vi "live_edited3.vi"() -> ()   [LabVIEW 2020]
uses:
  C:/Users/Public/Documents/Photometrics/PMQI-LabViewSamples/Examples/2018/Dependencies/PVCamNET.dll
  Dependencies/PVCamNET.dll
panel:
  in  "Full CCD Height":u16
  in  "Full CCD Width":u16
  in  "Full CCD":bool
  in  "Get ROI":bool
  in  "Height":u16
  in  "Y":u16
  in  "Width":u16
  in  "X":u16
  out "Trigger Mode":i32
  in  "Trigger In Behaviour":string(combo)
  out "Exp. out":i32
  in  "Trigger Out Behaviour":string(combo)
  out "Boolean":bool
  in  "Scan Direction Reset":bool
  out "Scan Line Time":dbl format="%#_14g"
  in  "Scan Width":dbl
  in  "Scan Line Delay":dbl
  in  "Scan Direction":string(combo)
  in  "Scan Mode":string(combo)
  in  "Exposure Time":dbl
  in  "Live":bool
  in  "Camera Status":bool
  in  "Uninit":bool
  in  "Live stop":bool
  in  "Live start":bool
  in  "Open":bool
  # "Description:\nThis code lets the user use programmable scan\n mode for live imaging.\n\nSteps to run:\n1. Click \"Run\"\n2. Click \"Open\"\n3. Enter Exposure Time\n4. Select Scan Mode. \n5. Set Scan Line Delay or Scan Width\n6. Select Scan Direction\n7. Click \"Live start\"\n8. Click \"Live stop\"\n9. Right click on CamWindow and add a ROI.\n10. Click \"Get ROI\"\n11. Click \"Live start\"\n12. Click \"Live stop\"\n13. Right click on CamWindow and delete a ROI.\n14. Click \"Close\""
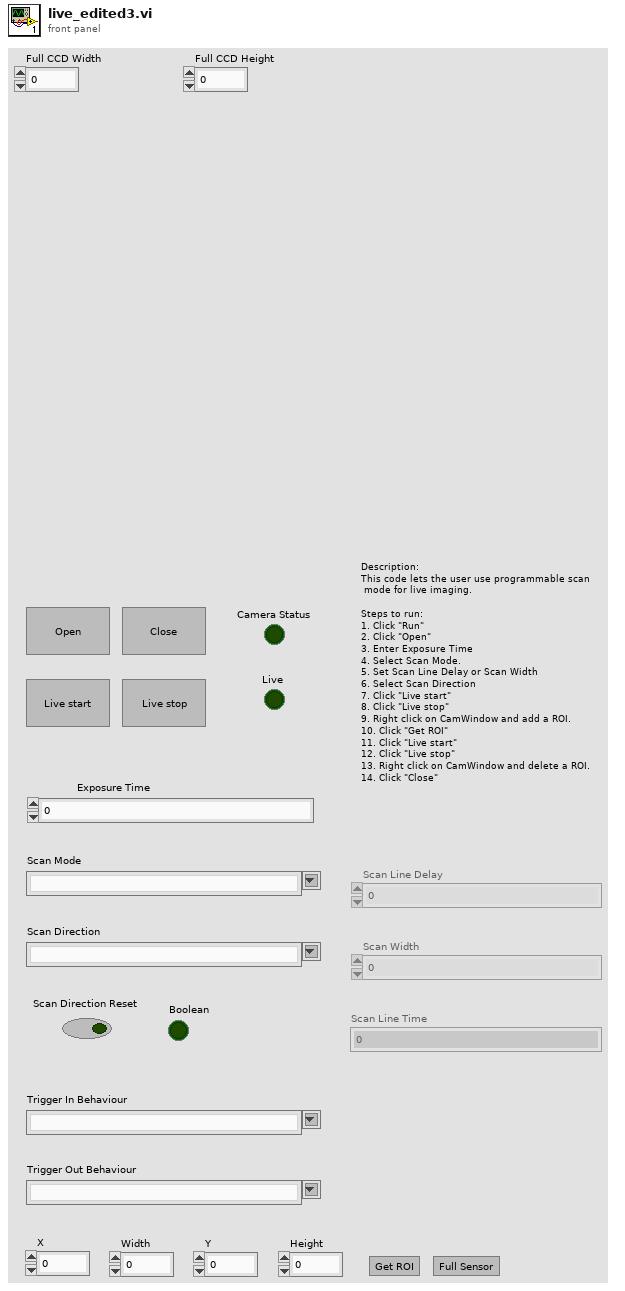
[diagram p1: front panel]
types:
  T1 = enum8{"Enabled", "Disabled", "Disabled and Grayed Out"}
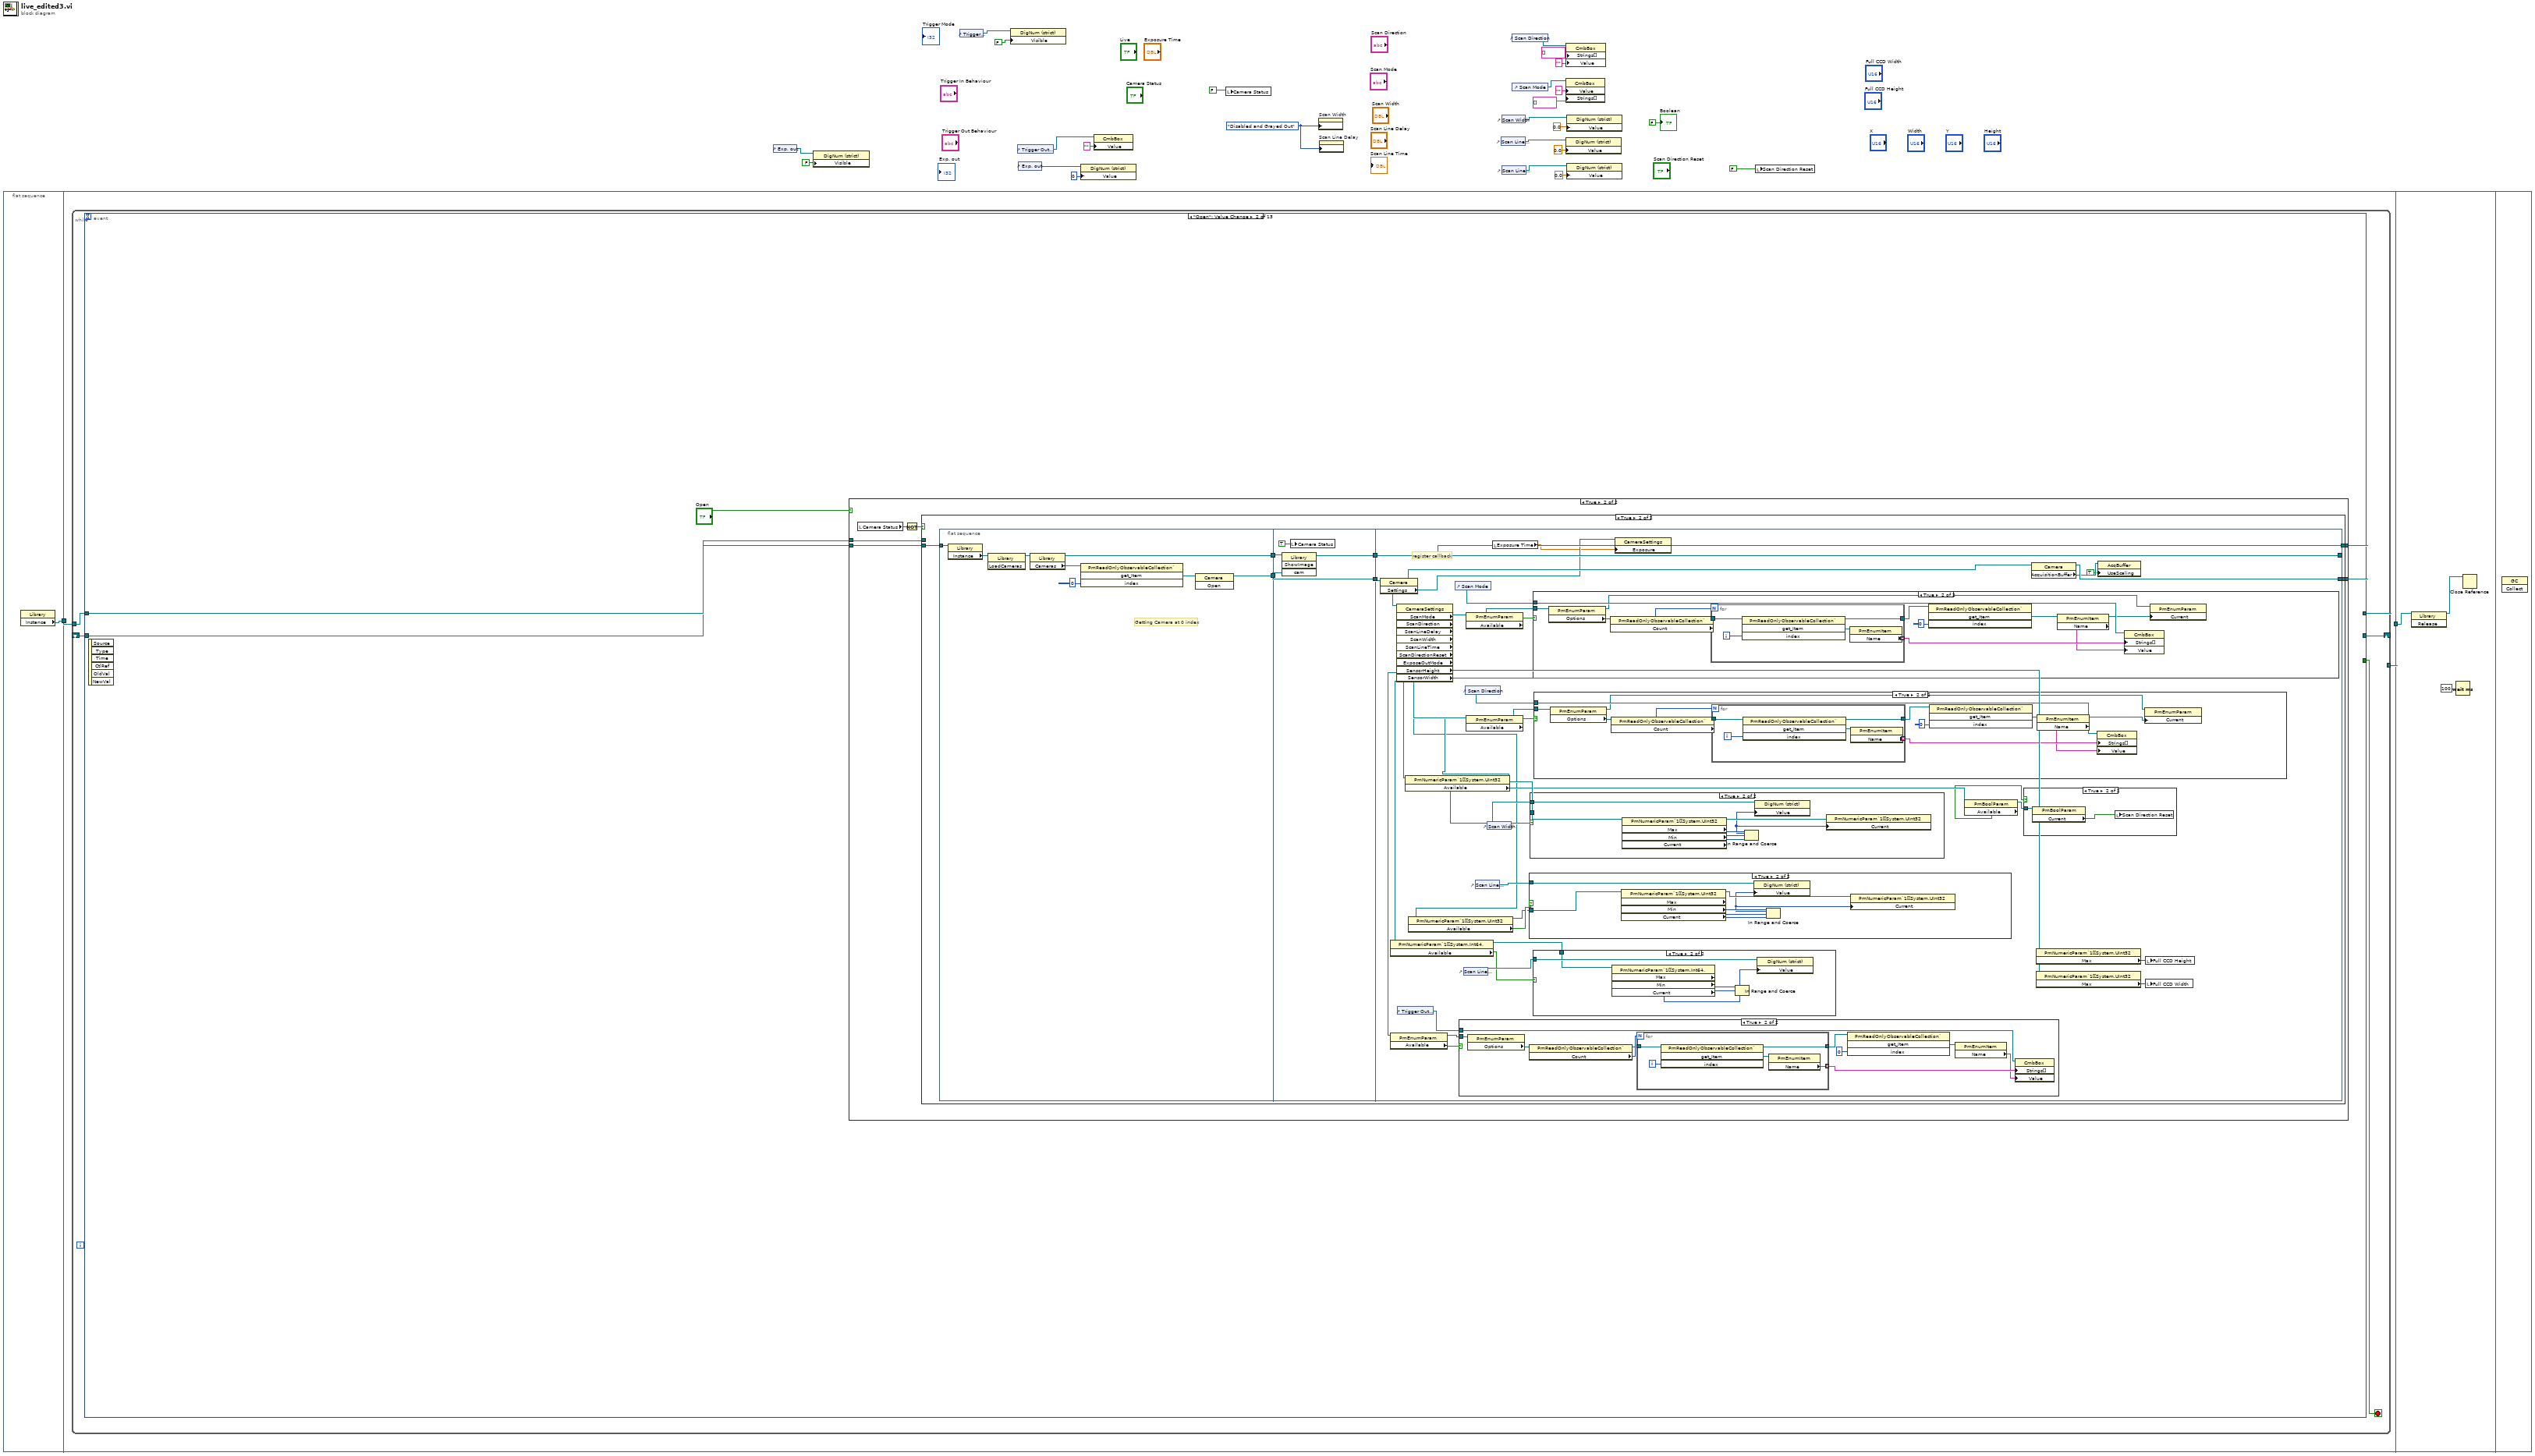
[diagram p0: block diagram]
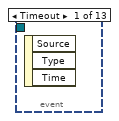
[diagram p2: hidden frame]
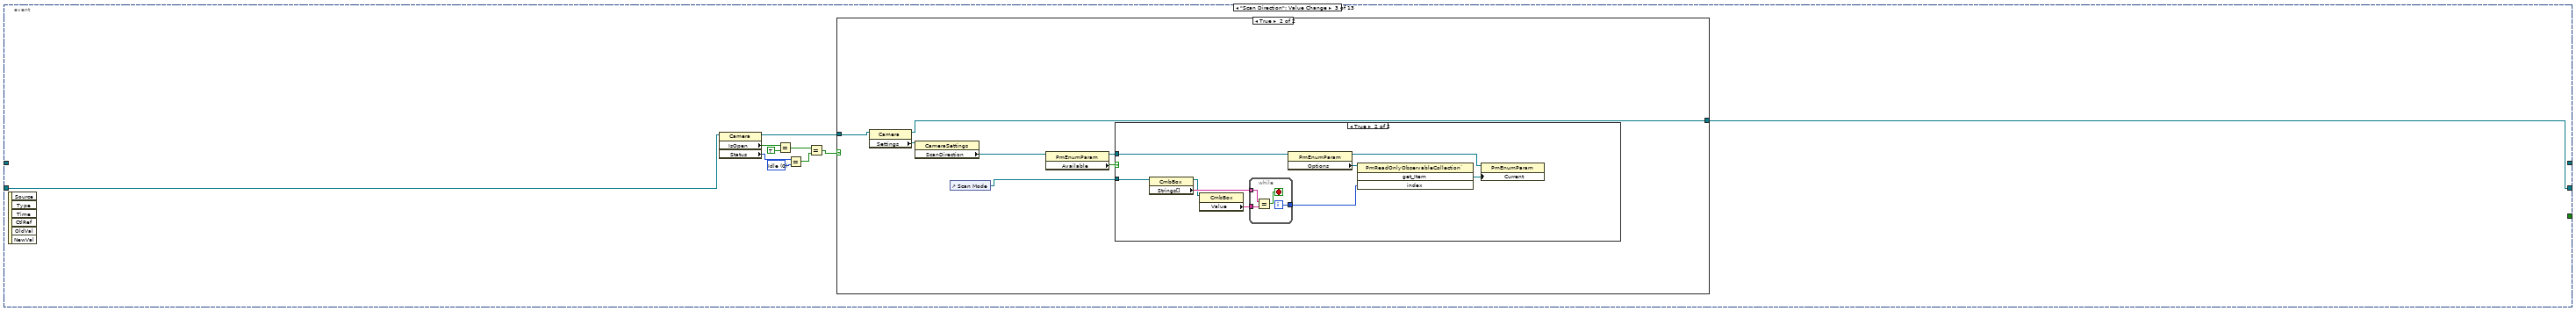
[diagram p12: hidden frame]
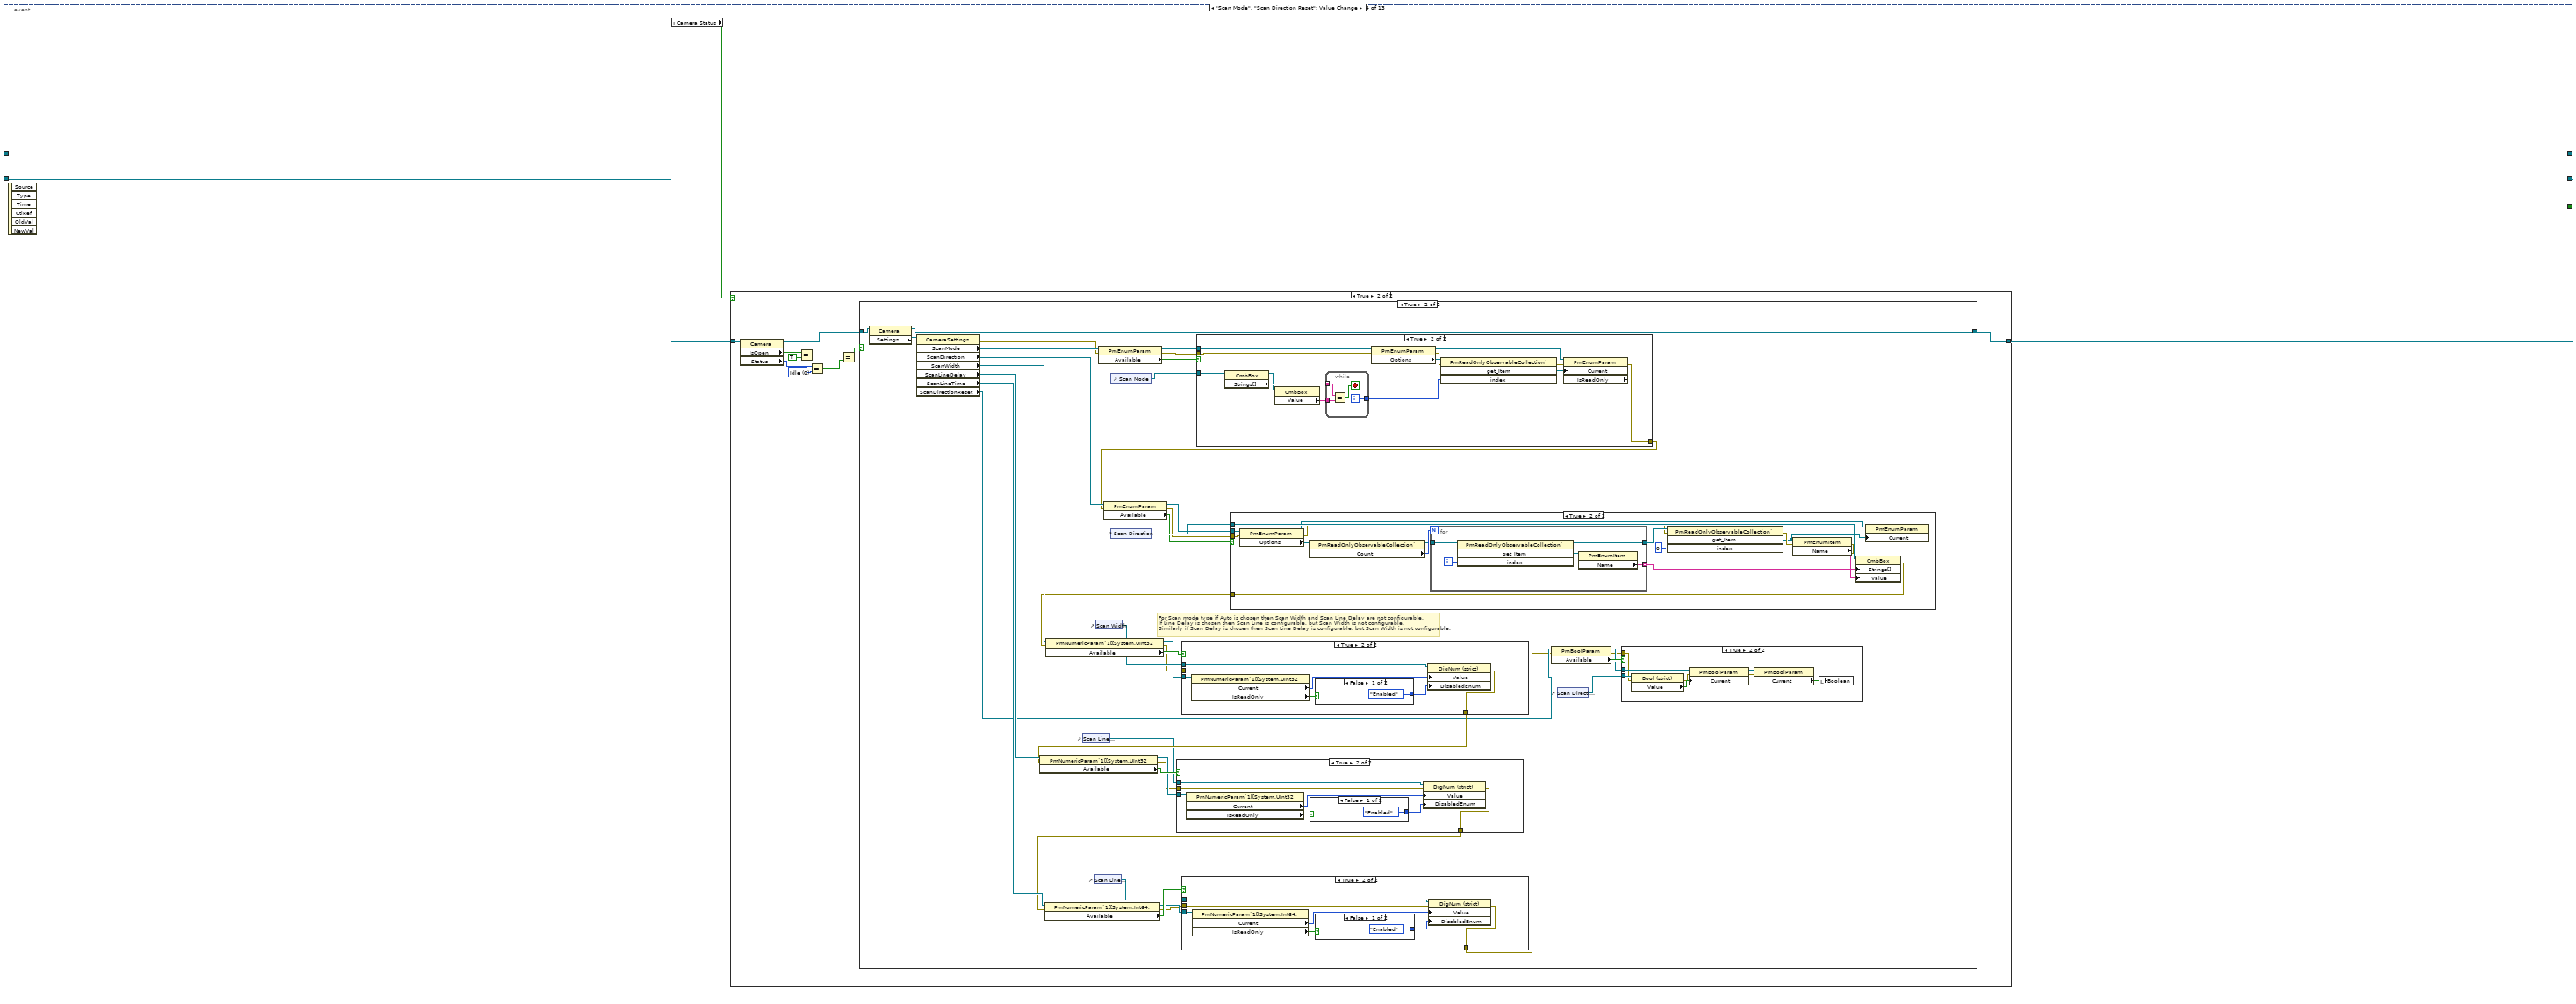
[diagram p15: hidden frame]
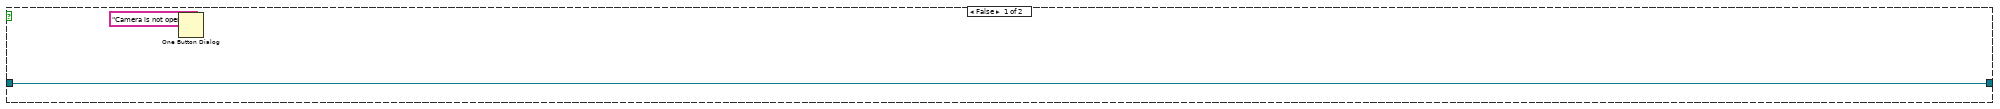
[diagram p16: hidden frame]
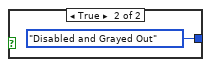
[diagram p20: hidden frame]
diagram:
  w11 = T1."Disabled and Grayed Out" ("Disabled")
  n1 = flat-sequence {
    tunnel: [w27] -> w26
    tunnel: w26 -> [w29]
    tunnel: [w28] -> w25
    tunnel: w25 -> [w765]
    frame #0 {
      n2 = property class="Library"() -> ("Instance"=w27:refnum<k24>)  [unwired: 2 in, 2 out]
    }
    frame #1 {
      n3 = while {
        tunnel: w29 -> [w34]
        shift-right: [w33] -> _
        shift-left: _ -> [w31]
        tunnel: [w32] -> w28
        stop <- w30 stop-if-true
        n4 = event shown="[1] \"Open\": Value Change" {
          selector: _ -> [_ _ _ _ _ _ _ _ _ _ _ _ _]
          dyn-events: _ -> [_ _ _ _ _ _ _ _ _ _ _ _ _]
          timeout: _ -> [_ _ _ _ _ _ _ _ _ _ _ _ _]
          tunnel: w34 -> [_ w39 _ _ _ _ w466 _ _ _ w682 _ w737]
          tunnel: [_ w38 w179 w211 w343 w407 w467 w534 w571 w644 w683 w712 w738] -> w33
          tunnel: [_ w37 _ _ _ _ w466 _ _ _ w682 _ w737] -> w32
          tunnel: w31 -> [_ w36 w183 w212 w349 w409 w468 w535 w572 w645 w684 w713 w739]
          tunnel: [_ _ _ _ _ _ _ _ _ _ _ _ w736] -> w30
          event Timeout {
            n5 = event-data() -> ()  [unwired: 1 in, 3 out]
          }
          event "Open": Value Change {
            n6 = event-data() -> ()  [unwired: 1 in, 6 out]
            n7 = case shown="True" "Open" {
              tunnel: w39 -> [w41 w47]
              tunnel: [w40 w46] -> w38
              tunnel: [w41 w45] -> w37
              tunnel: w36 -> [w40 w42]
              frame False {
              }
              frame True {
                n8 = local read "Camera Status"() -> (w44:bool)
                n9 = Not(x=w44) -> (.not. x?=w43:bool)
                n10 = case shown="True" w43 {
                  tunnel: w47 -> [w48 w54]
                  tunnel: [w49 w53] -> w46
                  tunnel: [w48 w52] -> w45
                  tunnel: w42 -> [w49 _]
                  frame False {
                  }
                  frame True {
                    n11 = flat-sequence {
                      tunnel: w54 -> [w59]
                      tunnel: [w61] -> w56
                      tunnel: [w60] -> w55
                      tunnel: w56 -> [w67]
                      tunnel: w55 -> [w68]
                      tunnel: [w68] -> w51
                      tunnel: [w66] -> w50
                      tunnel: [w107] -> w52
                      tunnel: [w87] -> w53
                      tunnel: w51 -> [w106]
                      tunnel: w50 -> [w107]
                      frame #0 {
                        # "Getting Camera at 0 index"
                        n12 = property class="Library"(reference=w59) -> ("Instance"=w58:refnum<k24>)  [unwired: 1 in, 2 out]
                        n13 = invoke class="Library" method="LoadCameras"(reference=w58) -> (reference out=w57:refnum<k24>)  [unwired: 2 in, 2 out]
                        n14 = property class="Library"(reference=w57) -> (reference out=w61:refnum<k24>, "Cameras"=w64:refnum<k24>)  [unwired: 1 in, 1 out]
                        n15 = invoke class="PmReadOnlyObservableCollection`" method="get_Item"(reference=w64, "index"=0) -> ("get_Item"=w62:refnum<k24>)  [unwired: 2 in, 3 out]
                        n16 = invoke class="Camera" method="Open"(reference=w62) -> (reference out=w60:refnum<k24>)  [unwired: 2 in, 2 out]
                      }
                      frame #1 {
                        n17 = invoke class="Library" method="ShowImage"(reference=w67, "cam"=w68) -> (reference out=w66:refnum<k24>)  [unwired: 2 in, 3 out]
                        n18 = local write "Camera Status"(TRUE ("Camera Status")) -> ()
                      }
                      frame #2 {
                        # "register callback"
                        n19 = property class="Camera"(reference=w106) -> (reference out=w88:refnum<k24>, "Settings"=w77:refnum<k24>)  [unwired: 1 in, 1 out]
                        n20 = property class="CameraSettings"(reference=w77) -> ("ScanMode"=w105:refnum<k24>, "ScanDirection"=w101:refnum<k24>, "ScanLineDelay"=w96:refnum<k24>, "ScanWidth"=w83:refnum<k24>, "ScanLineTime"=w75:refnum<k24>, "ScanDirectionReset"=w91:refnum<k24>, "ExposeOutMode"=w79:refnum<k24>, "SensorHeight"=w70:refnum<k24>, "SensorWidth"=w69:refnum<k24>)  [unwired: 1 in, 2 out]
                        n21 = property class="PmNumericParam`1[[System.Int64,"(reference=w75) -> (reference out=w73:refnum<k24>, "Available"=w74:bool)  [unwired: 1 in, 1 out]
                        n22 = property class="PmEnumParam"(reference=w79) -> (reference out=w80:refnum<k24>, "Available"=w81:bool)  [unwired: 1 in, 1 out]
                        n23 = control-ref of="Trigger Out Behaviour"() -> (w78:refnum<vi>)
                        n24 = property class="PmNumericParam`1[[System.UInt32"(reference=w96) -> (reference out=w94:refnum<k24>, "Available"=w95:bool)  [unwired: 1 in, 1 out]
                        n25 = property class="PmNumericParam`1[[System.UInt32"(reference=w83) -> (reference out=w82:refnum<k24>, "Available"=w84:bool)  [unwired: 1 in, 1 out]
                        n26 = control-ref of="Scan Mode"() -> (w102:refnum<vi>)
                        n27 = case shown="True" w81 {
                          tunnel: w80 -> [_ w117]
                          tunnel: w78 -> [_ w108]
                          frame False {
                          }
                          frame True {
                            n28 = property class="PmEnumParam"(reference=w117) -> ("Options"=w116:refnum<k24>)  [unwired: 1 in, 2 out]
                            n29 = property class="PmReadOnlyObservableCollection`"(reference=w116) -> (reference out=w114:refnum<k24>, "Count"=w115:i32)  [unwired: 1 in, 1 out]
                            n30 = for {
                              N: w115 -> [_]
                              tunnel: w114 -> [w122]
                              tunnel: [w119] -> w111
                              tunnel: [w118] -> w110 mode=indexing
                              i -> [w121]
                              n31 = invoke class="PmReadOnlyObservableCollection`" method="get_Item"(reference=w122, "index"=w121) -> (reference out=w119:refnum<k24>, "get_Item"=w120:refnum<k24>)  [unwired: 2 in, 2 out]
                              n32 = property class="PmEnumItem"(reference=w120) -> ("Name"=w118:string)  [unwired: 1 in, 2 out]
                            }
                            n33 = invoke class="PmReadOnlyObservableCollection`" method="get_Item"(reference=w111, "index"=0) -> ("get_Item"=w112:refnum<k24>)  [unwired: 2 in, 3 out]
                            n34 = property class="PmEnumItem"(reference=w112) -> ("Name"=w109:string)  [unwired: 1 in, 2 out]
                            n35 = property class="CmbBox"(reference=w108, "Strings[]"=w110, "Value"=w109) -> ()  [unwired: 1 in, 2 out]
                          }
                        }
                        n36 = control-ref of="Scan Line Time"() -> (w92:refnum<vi>)
                        n37 = control-ref of="Scan Direction"() -> (w98:refnum<vi>)
                        n38 = property class="PmEnumParam"(reference=w105) -> (reference out=w103:refnum<k24>, "Available"=w104:bool)  [unwired: 1 in, 1 out]
                        n39 = property class="PmEnumParam"(reference=w101) -> (reference out=w99:refnum<k24>, "Available"=w100:bool)  [unwired: 1 in, 1 out]
                        n40 = control-ref of="Scan Line Delay"() -> (w93:refnum<vi>)
                        n41 = control-ref of="Scan Width"() -> (w97:refnum<vi>)
                        n42 = local read "Exposure Time"() -> (w76:dbl)
                        n43 = case shown="True" w84 {
                          tunnel: w93 -> [_ w134]
                          tunnel: w82 -> [_ w133]
                          frame False {
                          }
                          frame True {
                            n44 = property class="PmNumericParam`1[[System.UInt32"(reference=w133) -> (reference out=w132:refnum<k24>, "Max"=w135:u32, "Min"=w136:u32, "Current"=w137:u32)  [unwired: 1 in, 1 out]
                            n45 = In Range and Coerce(upper limit=w135, x=w137, lower limit=w136) -> (coerced(x)=w131:u32)  [unwired: 1 out]
                            n46 = property class="DigNum (strict)"(reference=w134, "Value"=w131) -> ()  [unwired: 1 in, 2 out]
                            n47 = property class="PmNumericParam`1[[System.UInt32"(reference=w132, "Current"=w131) -> ()  [unwired: 1 in, 2 out]
                          }
                        }
                        n48 = case shown="True" w95 {
                          tunnel: w97 -> [_ w141]
                          tunnel: w94 -> [_ w140]
                          frame False {
                          }
                          frame True {
                            n49 = property class="PmNumericParam`1[[System.UInt32"(reference=w140) -> (reference out=w139:refnum<k24>, "Max"=w142:u32, "Min"=w143:u32, "Current"=w144:u32)  [unwired: 1 in, 1 out]
                            n50 = In Range and Coerce(upper limit=w142, x=w144, lower limit=w143) -> (coerced(x)=w138:u32)  [unwired: 1 out]
                            n51 = property class="DigNum (strict)"(reference=w141, "Value"=w138) -> ()  [unwired: 1 in, 2 out]
                            n52 = property class="PmNumericParam`1[[System.UInt32"(reference=w139, "Current"=w138) -> ()  [unwired: 1 in, 2 out]
                          }
                        }
                        n53 = case shown="True" w74 {
                          tunnel: w92 -> [_ w126]
                          tunnel: w73 -> [_ w125]
                          frame False {
                          }
                          frame True {
                            n54 = property class="PmNumericParam`1[[System.Int64,"(reference=w125) -> ("Max"=w127:i64, "Min"=w128:i64, "Current"=w129:i64)  [unwired: 1 in, 2 out]
                            n55 = In Range and Coerce(upper limit=w127, x=w129, lower limit=w128) -> (coerced(x)=w130:i64)  [unwired: 1 out]
                            n56 = property class="DigNum (strict)"(reference=w126, "Value"=w130) -> ()  [unwired: 1 in, 2 out]
                          }
                        }
                        n57 = case shown="True" w104 {
                          tunnel: w103 -> [_ w173]
                          tunnel: w102 -> [_ w165]
                          frame False {
                          }
                          frame True {
                            n58 = property class="PmEnumParam"(reference=w173) -> (reference out=w164:refnum<k24>, "Options"=w172:refnum<k24>)  [unwired: 1 in, 1 out]
                            n59 = property class="PmReadOnlyObservableCollection`"(reference=w172) -> (reference out=w170:refnum<k24>, "Count"=w171:i32)  [unwired: 1 in, 1 out]
                            n60 = for {
                              N: w171 -> [_]
                              tunnel: w170 -> [w178]
                              tunnel: [w175] -> w168
                              tunnel: [w174] -> w167 mode=indexing
                              i -> [w177]
                              n61 = invoke class="PmReadOnlyObservableCollection`" method="get_Item"(reference=w178, "index"=w177) -> (reference out=w175:refnum<k24>, "get_Item"=w176:refnum<k24>)  [unwired: 2 in, 2 out]
                              n62 = property class="PmEnumItem"(reference=w176) -> ("Name"=w174:string)  [unwired: 1 in, 2 out]
                            }
                            n63 = invoke class="PmReadOnlyObservableCollection`" method="get_Item"(reference=w168, "index"=0) -> ("get_Item"=w163:refnum<k24>)  [unwired: 2 in, 3 out]
                            n64 = property class="PmEnumItem"(reference=w163) -> (reference out=w162:refnum<k24>, "Name"=w166:string)  [unwired: 1 in, 1 out]
                            n65 = property class="CmbBox"(reference=w165, "Strings[]"=w167, "Value"=w166) -> ()  [unwired: 1 in, 2 out]
                            n66 = property class="PmEnumParam"(reference=w164, "Current"=w162) -> ()  [unwired: 1 in, 2 out]
                          }
                        }
                        n67 = case shown="True" w100 {
                          tunnel: w99 -> [_ w156]
                          tunnel: w98 -> [_ w147]
                          frame False {
                          }
                          frame True {
                            n68 = property class="PmEnumParam"(reference=w156) -> (reference out=w146:refnum<k24>, "Options"=w155:refnum<k24>)  [unwired: 1 in, 1 out]
                            n69 = property class="PmReadOnlyObservableCollection`"(reference=w155) -> (reference out=w153:refnum<k24>, "Count"=w154:i32)  [unwired: 1 in, 1 out]
                            n70 = for {
                              N: w154 -> [_]
                              tunnel: w153 -> [w161]
                              tunnel: [w158] -> w150
                              tunnel: [w157] -> w149 mode=indexing
                              i -> [w160]
                              n71 = invoke class="PmReadOnlyObservableCollection`" method="get_Item"(reference=w161, "index"=w160) -> (reference out=w158:refnum<k24>, "get_Item"=w159:refnum<k24>)  [unwired: 2 in, 2 out]
                              n72 = property class="PmEnumItem"(reference=w159) -> ("Name"=w157:string)  [unwired: 1 in, 2 out]
                            }
                            n73 = invoke class="PmReadOnlyObservableCollection`" method="get_Item"(reference=w150, "index"=0) -> ("get_Item"=w151:refnum<k24>)  [unwired: 2 in, 3 out]
                            n74 = property class="PmEnumItem"(reference=w151) -> (reference out=w145:refnum<k24>, "Name"=w148:string)  [unwired: 1 in, 1 out]
                            n75 = property class="CmbBox"(reference=w147, "Strings[]"=w149, "Value"=w148) -> ()  [unwired: 1 in, 2 out]
                            n76 = property class="PmEnumParam"(reference=w146, "Current"=w145) -> ()  [unwired: 1 in, 2 out]
                          }
                        }
                        n77 = property class="CameraSettings"(reference=w77, "Exposure"=w76) -> ()  [unwired: 1 in, 2 out]
                        n78 = property class="PmBoolParam"(reference=w91) -> (reference out=w89:refnum<k24>, "Available"=w90:bool)  [unwired: 1 in, 1 out]
                        n79 = case shown="True" w90 {
                          tunnel: w89 -> [_ w124]
                          frame False {
                          }
                          frame True {
                            n80 = property class="PmBoolParam"(reference=w124) -> ("Current"=w123:bool)  [unwired: 1 in, 2 out]
                            n81 = local write "Scan Direction Reset"(w123) -> ()
                          }
                        }
                        n82 = property class="Camera"(reference=w88) -> (reference out=w87:refnum<k24>, "AcquisitionBuffer"=w86:refnum<k24>)  [unwired: 1 in, 1 out]
                        n83 = property class="PmNumericParam`1[[System.UInt32"(reference=w70) -> ("Max"=w72:u32)  [unwired: 1 in, 2 out]
                        n84 = property class="PmNumericParam`1[[System.UInt32"(reference=w69) -> ("Max"=w71:u32)  [unwired: 1 in, 2 out]
                        n85 = property class="AcqBuffer"(reference=w86, "UseScaling"=TRUE) -> ()  [unwired: 1 in, 2 out]
                        n86 = local write "Full CCD Height"(w72) -> ()
                        n87 = local write "Full CCD Width"(w71) -> ()
                      }
                    }
                  }
                }
              }
            }
          }
          event "Scan Direction": Value Change {
            w187 = 0 items=["Idle", "Capturing"] ("Status")
            n88 = event-data() -> ()  [unwired: 1 in, 6 out]
            n89 = property class="Camera"(reference=w183) -> (reference out=w180:refnum<k24>, "IsOpen"=w186:bool, "Status"=w188:i32)  [unwired: 1 in, 1 out]
            n90 = Equal?(x=w186, y=TRUE) -> (x = y?=w182:bool)
            n91 = Equal?(x=w188, y=w187) -> (x = y?=w184:bool)
            n92 = Equal?(x=w182, y=w184) -> (x = y?=w181:bool)
            n93 = case shown="True" w181 {
              tunnel: w180 -> [w189 w193]
              tunnel: [w189 w190] -> w179
              frame False {
              }
              frame True {
                n94 = property class="Camera"(reference=w193) -> (reference out=w190:refnum<k24>, "Settings"=w194:refnum<k24>)  [unwired: 1 in, 1 out]
                n95 = property class="CameraSettings"(reference=w194) -> ("ScanDirection"=w192:refnum<k24>)  [unwired: 1 in, 2 out]
                n96 = control-ref of="Scan Mode"() -> (w191:refnum<vi>)
                n97 = property class="PmEnumParam"(reference=w192) -> (reference out=w195:refnum<k24>, "Available"=w196:bool)  [unwired: 1 in, 1 out]
                n98 = case shown="True" w196 {
                  tunnel: w195 -> [_ w204]
                  tunnel: w191 -> [_ w197]
                  frame False {
                  }
                  frame True {
                    n99 = property class="CmbBox"(reference=w197) -> (reference out=w199:refnum<vi>, "Strings[]"=w205:string[])  [unwired: 1 in, 1 out]
                    n100 = property class="CmbBox"(reference=w199) -> ("Value"=w198:string)  [unwired: 1 in, 2 out]
                    n101 = while {
                      tunnel: w205 -> [w209] mode=indexing
                      tunnel: [w207] -> w202
                      tunnel: w198 -> [w206]
                      i -> [w207]
                      stop <- w208 stop-if-true
                      n102 = Equal?(x=w209, y=w206) -> (x = y?=w208:bool)
                    }
                    n103 = property class="PmEnumParam"(reference=w204) -> (reference out=w201:refnum<k24>, "Options"=w203:refnum<k24>)  [unwired: 1 in, 1 out]
                    n104 = invoke class="PmReadOnlyObservableCollection`" method="get_Item"(reference=w203, "index"=w202) -> ("get_Item"=w200:refnum<k24>)  [unwired: 2 in, 3 out]
                    n105 = property class="PmEnumParam"(reference=w201, "Current"=w200) -> ()  [unwired: 1 in, 2 out]
                  }
                }
              }
            }
          }
          event "Scan Mode", "Scan Direction Reset": Value Change {
            n106 = event-data() -> ()  [unwired: 1 in, 6 out]
            n107 = local read "Camera Status"() -> (w210:bool)
            n108 = case shown="True" w210 {
              tunnel: w212 -> [w213 w218]
              tunnel: [w213 w216] -> w211
              frame False {
                n109 = One Button Dialog(message="Camera is not open") -> ()  [unwired: 1 in, 1 out]
              }
              frame True {
                w223 = 0 items=["Idle", "Capturing"] ("Status")
                n110 = property class="Camera"(reference=w218) -> (reference out=w217:refnum<k24>, "IsOpen"=w222:bool, "Status"=w224:i32)  [unwired: 1 in, 1 out]
                n111 = Equal?(x=w222, y=TRUE) -> (x = y?=w220:bool)
                n112 = Equal?(x=w224, y=w223) -> (x = y?=w219:bool)
                n113 = Equal?(x=w220, y=w219) -> (x = y?=w215:bool)
                n114 = case shown="True" w215 {
                  tunnel: w217 -> [w225 w264]
                  tunnel: [w225 w259] -> w216
                  frame False {
                  }
                  frame True {
                    # "For Scan mode type if Auto is chosen then Scan Width and Scan Line Delay are not configurable.\nIf Line Delay is chosen then Scan Line is configurable, but Scan Width is not configurable.\nSimilarly if Scan Delay is chosen then Scan Line Delay is configurable, but Scan Width is not configurable."
                    n115 = property class="Camera"(reference=w264) -> (reference out=w259:refnum<k24>, "Settings"=w263:refnum<k24>)  [unwired: 1 in, 1 out]
                    n116 = property class="CameraSettings"(reference=w263) -> (error out=w256:errorcluster, "ScanMode"=w262:refnum<k24>, "ScanDirection"=w258:refnum<k24>, "ScanWidth"=w254:refnum<k24>, "ScanLineDelay"=w253:refnum<k24>, "ScanLineTime"=w242:refnum<k24>, "ScanDirectionReset"=w231:refnum<k24>)  [unwired: 1 in, 1 out]
                    n117 = control-ref of="Scan Line Delay"() -> (w233:refnum<vi>)
                    n118 = control-ref of="Scan Line Time"() -> (w236:refnum<vi>)
                    n119 = control-ref of="Scan Width"() -> (w249:refnum<vi>)
                    n120 = property class="PmEnumParam"(reference=w262, error in=w256) -> (reference out=w260:refnum<k24>, error out=w257:errorcluster, "Available"=w261:bool)
                    n121 = control-ref of="Scan Mode"() -> (w255:refnum<vi>)
                    n122 = control-ref of="Scan Direction"() -> (w252:refnum<vi>)
                    n123 = case shown="True" w261 {
                      tunnel: w260 -> [_ w337]
                      tunnel: w255 -> [_ w332]
                      tunnel: w257 -> [w325 w331]
                      tunnel: [w325 w326] -> w241
                      frame False {
                      }
                      frame True {
                        n124 = property class="CmbBox"(reference=w332) -> (reference out=w333:refnum<vi>, "Strings[]"=w338:string[])  [unwired: 1 in, 1 out]
                        n125 = property class="CmbBox"(reference=w333) -> ("Value"=w328:string)  [unwired: 1 in, 2 out]
                        n126 = while {
                          tunnel: w338 -> [w342] mode=indexing
                          tunnel: [w340] -> w335
                          tunnel: w328 -> [w339]
                          i -> [w340]
                          stop <- w341 stop-if-true
                          n127 = Equal?(x=w342, y=w339) -> (x = y?=w341:bool)
                        }
                        n128 = property class="PmEnumParam"(reference=w337, error in=w331) -> (reference out=w334:refnum<k24>, error out=w330:errorcluster, "Options"=w336:refnum<k24>)
                        n129 = invoke class="PmReadOnlyObservableCollection`" method="get_Item"(reference=w336, error in=w330, "index"=w335) -> (error out=w329:errorcluster, "get_Item"=w327:refnum<k24>)  [unwired: 1 in, 2 out]
                        n130 = property class="PmEnumParam" props=["Current", "IsReadOnly"](reference=w334, error in=w329, "Current"=w327) -> (error out=w326:errorcluster)  [unwired: 2 out]
                      }
                    }
                    n131 = property class="PmEnumParam"(reference=w258, error in=w241) -> (reference out=w250:refnum<k24>, error out=w244:errorcluster, "Available"=w251:bool)
                    n132 = case shown="True" w251 {
                      tunnel: w250 -> [_ w319]
                      tunnel: w252 -> [_ w311]
                      tunnel: w244 -> [w303 w310]
                      tunnel: [w303 w304] -> w243
                      frame False {
                      }
                      frame True {
                        n133 = property class="PmEnumParam"(reference=w319, error in=w310) -> (reference out=w305:refnum<k24>, error out=w309:errorcluster, "Options"=w318:refnum<k24>)
                        n134 = property class="PmReadOnlyObservableCollection`"(reference=w318) -> (reference out=w316:refnum<k24>, "Count"=w317:i32)  [unwired: 1 in, 1 out]
                        n135 = for {
                          N: w317 -> [_]
                          tunnel: w316 -> [w324]
                          tunnel: [w321] -> w314
                          tunnel: [w320] -> w313 mode=indexing
                          i -> [w323]
                          n136 = invoke class="PmReadOnlyObservableCollection`" method="get_Item"(reference=w324, "index"=w323) -> (reference out=w321:refnum<k24>, "get_Item"=w322:refnum<k24>)  [unwired: 2 in, 2 out]
                          n137 = property class="PmEnumItem"(reference=w322) -> ("Name"=w320:string)  [unwired: 1 in, 2 out]
                        }
                        n138 = invoke class="PmReadOnlyObservableCollection`" method="get_Item"(reference=w314, error in=w309, "index"=0) -> (error out=w308:errorcluster, "get_Item"=w306:refnum<k24>)  [unwired: 1 in, 2 out]
                        n139 = property class="PmEnumItem"(reference=w306, error in=w308) -> (error out=w307:errorcluster, "Name"=w312:string)  [unwired: 1 out]
                        n140 = property class="CmbBox"(reference=w311, error in=w307, "Strings[]"=w313, "Value"=w312) -> (error out=w304:errorcluster)  [unwired: 1 out]
                        n141 = property class="PmEnumParam"(reference=w305, "Current"=w306) -> ()  [unwired: 1 in, 2 out]
                      }
                    }
                    n142 = property class="PmNumericParam`1[[System.UInt32"(reference=w254, error in=w243) -> (reference out=w247:refnum<k24>, error out=w246:errorcluster, "Available"=w248:bool)
                    n143 = case shown="True" w248 {
                      tunnel: w249 -> [_ w299]
                      tunnel: w247 -> [_ w296]
                      tunnel: w246 -> [w293 w298]
                      tunnel: [w293 w297] -> w245
                      frame False {
                      }
                      frame True {
                        n144 = property class="PmNumericParam`1[[System.UInt32"(reference=w296) -> ("Current"=w300:u32, "IsReadOnly"=w295:bool)  [unwired: 1 in, 2 out]
                        n145 = case shown="False" w295 {
                          tunnel: [T1."Enabled" ("Disabled") T1."Disabled and Grayed Out" ("Disabled")] -> w294
                          frame False {
                          }
                          frame True {
                          }
                        }
                        n146 = property class="DigNum (strict)"(reference=w299, error in=w298, "Value"=w300, "DisabledEnum"=w294) -> (error out=w297:errorcluster)  [unwired: 1 out]
                      }
                    }
                    n147 = property class="PmNumericParam`1[[System.UInt32"(reference=w253, error in=w245) -> (reference out=w238:refnum<k24>, error out=w232:errorcluster, "Available"=w239:bool)
                    n148 = case shown="True" w239 {
                      tunnel: w233 -> [_ w289]
                      tunnel: w238 -> [_ w286]
                      tunnel: w232 -> [w283 w288]
                      tunnel: [w283 w287] -> w235
                      frame False {
                      }
                      frame True {
                        n149 = property class="PmNumericParam`1[[System.UInt32"(reference=w286) -> ("Current"=w290:u32, "IsReadOnly"=w285:bool)  [unwired: 1 in, 2 out]
                        n150 = case shown="False" w285 {
                          tunnel: [T1."Enabled" ("Disabled") T1."Disabled and Grayed Out" ("Disabled")] -> w284
                          frame False {
                          }
                          frame True {
                          }
                        }
                        n151 = property class="DigNum (strict)"(reference=w289, error in=w288, "Value"=w290, "DisabledEnum"=w284) -> (error out=w287:errorcluster)  [unwired: 1 out]
                      }
                    }
                    n152 = property class="PmNumericParam`1[[System.Int64,"(reference=w242, error in=w235) -> (reference out=w237:refnum<k24>, error out=w234:errorcluster, "Available"=w240:bool)
                    n153 = case shown="True" w240 {
                      tunnel: w236 -> [_ w279]
                      tunnel: w237 -> [_ w276]
                      tunnel: w234 -> [w273 w278]
                      tunnel: [w273 w277] -> w227
                      frame False {
                      }
                      frame True {
                        n154 = property class="PmNumericParam`1[[System.Int64,"(reference=w276) -> ("Current"=w280:i64, "IsReadOnly"=w275:bool)  [unwired: 1 in, 2 out]
                        n155 = case shown="False" w275 {
                          tunnel: [T1."Enabled" ("Disabled") T1."Disabled and Grayed Out" ("Disabled")] -> w274
                          frame False {
                          }
                          frame True {
                          }
                        }
                        n156 = property class="DigNum (strict)"(reference=w279, error in=w278, "Value"=w280, "DisabledEnum"=w274) -> (error out=w277:errorcluster)  [unwired: 1 out]
                      }
                    }
                    n157 = property class="PmBoolParam"(reference=w231, error in=w227) -> (reference out=w229:refnum<k24>, error out=w226:errorcluster, "Available"=w230:bool)
                    n158 = control-ref of="Scan Direction Reset"() -> (w228:refnum<vi>)
                    n159 = case shown="True" w230 {
                      tunnel: w229 -> [_ w270]
                      tunnel: w228 -> [_ w272]
                      tunnel: w226 -> [_ w267]
                      frame False {
                      }
                      frame True {
                        n160 = property class="Bool (strict)"(reference=w272, error in=w267) -> (error out=w266:errorcluster, "Value"=w271:bool)  [unwired: 1 out]
                        n161 = property class="PmBoolParam"(reference=w270, error in=w266, "Current"=w271) -> (reference out=w269:refnum<k24>, error out=w265:errorcluster)
                        n162 = property class="PmBoolParam"(reference=w269, error in=w265) -> ("Current"=w268:bool)  [unwired: 2 out]
                        n163 = local write "Boolean"(w268) -> ()
                      }
                    }
                  }
                }
              }
            }
          }
          event "Scan Line Delay": Value Change {
            w354 = 0 items=["Idle", "Capturing"] ("Status")
            n164 = event-data() -> ()  [unwired: 1 in, 6 out]
            n165 = property class="Camera"(reference=w349) -> (reference out=w348:refnum<k24>, "IsOpen"=w353:bool, "Status"=w355:i32)  [unwired: 1 in, 1 out]
            n166 = Equal?(x=w353, y=TRUE) -> (x = y?=w351:bool)
            n167 = Equal?(x=w355, y=w354) -> (x = y?=w350:bool)
            n168 = Equal?(x=w351, y=w350) -> (x = y?=w347:bool)
            n169 = control-ref of="Scan Line Time"() -> (w344:refnum<vi>)
            n170 = control-ref of="Scan Line Delay"() -> (w345:refnum<vi>)
            n171 = control-ref of="Scan Width"() -> (w346:refnum<vi>)
            n172 = case shown="True" w347 {
              tunnel: w348 -> [w356 w378]
              tunnel: [w356 w377] -> w343
              tunnel: w345 -> [_ w376]
              tunnel: w346 -> [_ w375]
              tunnel: w344 -> [_ w359]
              frame False {
              }
              frame True {
                n173 = property class="Camera"(reference=w378) -> (reference out=w377:refnum<k24>, "Settings"=w374:refnum<k24>)  [unwired: 1 in, 1 out]
                n174 = property class="CameraSettings"(reference=w374) -> (reference out=w364:refnum<k24>, error out=w370:errorcluster, "ScanLineDelay"=w373:refnum<k24>)  [unwired: 1 in]
                n175 = property class="PmNumericParam`1[[System.UInt32"(reference=w373, error in=w370) -> (reference out=w371:refnum<k24>, error out=w369:errorcluster, "Available"=w372:bool)
                n176 = case shown="True" w372 {
                  tunnel: w376 -> [_ w395]
                  tunnel: w371 -> [_ w394]
                  tunnel: w369 -> [w390 w393]
                  tunnel: [w390 w391] -> w365
                  frame False {
                  }
                  frame True {
                    n177 = property class="PmNumericParam`1[[System.UInt32"(reference=w394) -> (reference out=w398:refnum<k24>, "Max"=w396:u32, "Min"=w397:u32)  [unwired: 1 in, 1 out]
                    n178 = property class="DigNum (strict)"(reference=w395, error in=w393) -> (reference out=w402:refnum<vi>, error out=w392:errorcluster, "Value"=w401:dbl)
                    n179 = In Range and Coerce(upper limit=w396, x=w401, lower limit=w397) -> (coerced(x)=w400:dbl)  [unwired: 1 out]
                    n180 = property class="PmNumericParam`1[[System.UInt32"(reference=w398, "Current"=w400) -> (reference out=w399:refnum<k24>)  [unwired: 1 in, 1 out]
                    n181 = property class="PmNumericParam`1[[System.UInt32"(reference=w399) -> ("Current"=w403:u32)  [unwired: 1 in, 2 out]
                    n182 = property class="DigNum (strict)"(reference=w402, error in=w392, "Value"=w403) -> (error out=w391:errorcluster)  [unwired: 1 out]
                  }
                }
                n183 = property class="CameraSettings"(reference=w364) -> ("ScanWidth"=w363:refnum<k24>, "ScanLineTime"=w362:refnum<k24>)  [unwired: 1 in, 2 out]
                n184 = property class="PmNumericParam`1[[System.UInt32"(reference=w363, error in=w365) -> (reference out=w367:refnum<k24>, error out=w366:errorcluster, "Available"=w368:bool)
                n185 = case shown="True" w368 {
                  tunnel: w375 -> [_ w386]
                  tunnel: w367 -> [_ w389]
                  tunnel: w366 -> [w384 w387]
                  tunnel: [w384 w388] -> w358
                  frame False {
                  }
                  frame True {
                    n186 = property class="PmNumericParam`1[[System.UInt32"(reference=w389) -> ("Current"=w385:u32)  [unwired: 1 in, 2 out]
                    n187 = property class="DigNum (strict)"(reference=w386, error in=w387, "Value"=w385) -> (error out=w388:errorcluster)  [unwired: 1 out]
                  }
                }
                n188 = property class="PmNumericParam`1[[System.Int64,"(reference=w362, error in=w358) -> (reference out=w360:refnum<k24>, error out=w357:errorcluster, "Available"=w361:bool)
                n189 = case shown="True" w361 {
                  tunnel: w360 -> [_ w383]
                  tunnel: w359 -> [_ w381]
                  tunnel: w357 -> [_ w380]
                  frame False {
                  }
                  frame True {
                    n190 = property class="PmNumericParam`1[[System.Int64,"(reference=w383, error in=w380) -> (error out=w379:errorcluster, "Current"=w382:i64)  [unwired: 1 out]
                    n191 = property class="DigNum (strict)"(reference=w381, error in=w379, "Value"=w382) -> ()  [unwired: 2 out]
                  }
                }
              }
            }
          }
          event "Scan Width": Value Change {
            w415 = 0 items=["Idle", "Capturing"] ("Status")
            n192 = event-data() -> ()  [unwired: 1 in, 6 out]
            n193 = property class="Camera"(reference=w409) -> (reference out=w408:refnum<k24>, "IsOpen"=w414:bool, "Status"=w416:i32)  [unwired: 1 in, 1 out]
            n194 = Equal?(x=w414, y=TRUE) -> (x = y?=w412:bool)
            n195 = Equal?(x=w416, y=w415) -> (x = y?=w411:bool)
            n196 = Equal?(x=w412, y=w411) -> (x = y?=w410:bool)
            n197 = control-ref of="Scan Line Time"() -> (w404:refnum<vi>)
            n198 = control-ref of="Scan Width"() -> (w406:refnum<vi>)
            n199 = control-ref of="Scan Line Delay"() -> (w405:refnum<vi>)
            n200 = case shown="True" w410 {
              tunnel: w408 -> [w417 w439]
              tunnel: [w417 w438] -> w407
              tunnel: w406 -> [_ w437]
              tunnel: w405 -> [_ w436]
              tunnel: w404 -> [_ w421]
              frame False {
              }
              frame True {
                n201 = property class="Camera"(reference=w439) -> (reference out=w438:refnum<k24>, "Settings"=w435:refnum<k24>)  [unwired: 1 in, 1 out]
                n202 = property class="CameraSettings"(reference=w435) -> (reference out=w418:refnum<k24>, error out=w431:errorcluster, "ScanWidth"=w434:refnum<k24>)  [unwired: 1 in]
                n203 = property class="PmNumericParam`1[[System.UInt32"(reference=w434, error in=w431) -> (reference out=w432:refnum<k24>, error out=w430:errorcluster, "Available"=w433:bool)
                n204 = case shown="True" w433 {
                  tunnel: w437 -> [_ w456]
                  tunnel: w432 -> [_ w455]
                  tunnel: w430 -> [w451 w454]
                  tunnel: [w451 w452] -> w426
                  frame False {
                  }
                  frame True {
                    n205 = property class="PmNumericParam`1[[System.UInt32"(reference=w455) -> (reference out=w459:refnum<k24>, "Max"=w457:u32, "Min"=w458:u32)  [unwired: 1 in, 1 out]
                    n206 = property class="DigNum (strict)"(reference=w456, error in=w454) -> (reference out=w463:refnum<vi>, error out=w453:errorcluster, "Value"=w462:dbl)
                    n207 = In Range and Coerce(upper limit=w457, x=w462, lower limit=w458) -> (coerced(x)=w461:dbl)  [unwired: 1 out]
                    n208 = property class="PmNumericParam`1[[System.UInt32"(reference=w459, "Current"=w461) -> (reference out=w460:refnum<k24>)  [unwired: 1 in, 1 out]
                    n209 = property class="PmNumericParam`1[[System.UInt32"(reference=w460) -> ("Current"=w464:u32)  [unwired: 1 in, 2 out]
                    n210 = property class="DigNum (strict)"(reference=w463, error in=w453, "Value"=w464) -> (error out=w452:errorcluster)  [unwired: 1 out]
                  }
                }
                n211 = property class="CameraSettings"(reference=w418) -> ("ScanLineDelay"=w425:refnum<k24>, "ScanLineTime"=w424:refnum<k24>)  [unwired: 1 in, 2 out]
                n212 = property class="PmNumericParam`1[[System.UInt32"(reference=w425, error in=w426) -> (reference out=w428:refnum<k24>, error out=w427:errorcluster, "Available"=w429:bool)
                n213 = case shown="True" w429 {
                  tunnel: w436 -> [_ w447]
                  tunnel: w428 -> [_ w450]
                  tunnel: w427 -> [w445 w448]
                  tunnel: [w445 w449] -> w420
                  frame False {
                  }
                  frame True {
                    n214 = property class="PmNumericParam`1[[System.UInt32"(reference=w450) -> ("Current"=w446:u32)  [unwired: 1 in, 2 out]
                    n215 = property class="DigNum (strict)"(reference=w447, error in=w448, "Value"=w446) -> (error out=w449:errorcluster)  [unwired: 1 out]
                  }
                }
                n216 = property class="PmNumericParam`1[[System.Int64,"(reference=w424, error in=w420) -> (reference out=w422:refnum<k24>, error out=w419:errorcluster, "Available"=w423:bool)
                n217 = case shown="True" w423 {
                  tunnel: w422 -> [_ w444]
                  tunnel: w421 -> [_ w442]
                  tunnel: w419 -> [_ w441]
                  frame False {
                  }
                  frame True {
                    n218 = property class="PmNumericParam`1[[System.Int64,"(reference=w444, error in=w441) -> (error out=w440:errorcluster, "Current"=w443:i64)  [unwired: 1 out]
                    n219 = property class="DigNum (strict)"(reference=w442, error in=w440, "Value"=w443) -> ()  [unwired: 2 out]
                  }
                }
              }
            }
          }
          event "Trigger In Behaviour", "Trigger Out Behaviour": Value Change {
            n220 = event-data() -> ()  [unwired: 1 in, 6 out]
            n221 = local read "Camera Status"() -> (w465:bool)
            n222 = case shown="True" w465 {
              tunnel: w468 -> [w470 w474]
              tunnel: [w470 w471] -> w467
              frame False {
                n223 = One Button Dialog(message="Camera is not open") -> ()  [unwired: 1 in, 1 out]
              }
              frame True {
                w479 = 0 items=["Idle", "Capturing"] ("Status")
                n224 = property class="Camera"(reference=w474) -> (reference out=w472:refnum<k24>, "IsOpen"=w478:bool, "Status"=w480:i32)  [unwired: 1 in, 1 out]
                n225 = Equal?(x=w478, y=TRUE) -> (x = y?=w476:bool)
                n226 = Equal?(x=w480, y=w479) -> (x = y?=w475:bool)
                n227 = Equal?(x=w476, y=w475) -> (x = y?=w473:bool)
                n228 = case shown="True" w473 {
                  tunnel: w472 -> [w481 w503]
                  tunnel: [w481 w495] -> w471
                  frame False {
                  }
                  frame True {
                    n229 = property class="Camera"(reference=w503) -> (reference out=w495:refnum<k24>, "Settings"=w490:refnum<k24>)  [unwired: 1 in, 1 out]
                    n230 = control-ref of="Trigger In Behaviour"() -> (w485:refnum<vi>)
                    n231 = control-ref of="Trigger Mode"() -> (w486:refnum<vi>)
                    n232 = control-ref of="Trigger Out Behaviour"() -> (w491:refnum<vi>)
                    n233 = control-ref of="Exp. out"() -> (w492:refnum<vi>)
                    n234 = property class="CameraSettings"(reference=w490) -> (reference out=w489:refnum<k24>, "ExposureTime"=w488:refnum<k24>, "ExposureMode"=w482:refnum<k24>, "ExposeOutMode"=w487:refnum<k24>)  [unwired: 1 in, 1 out]
                    n235 = property class="PmEnumParam"(reference=w487) -> (reference out=w493:refnum<k24>, "Available"=w494:bool)  [unwired: 1 in, 1 out]
                    n236 = property class="PmEnumParam"(reference=w482) -> (reference out=w484:refnum<k24>, "Available"=w483:bool)  [unwired: 1 in, 1 out]
                    n237 = property class="PmNumericParam`1[[System.UInt64"(reference=w488) -> (reference out=w500:refnum<k24>, "Max"=w502:u64, "Min"=w501:u64)  [unwired: 1 in, 1 out]
                    n238 = case shown="True" w494 {
                      tunnel: w493 -> [_ w528]
                      tunnel: w492 -> [_ w522]
                      tunnel: w491 -> [_ w519]
                      frame False {
                      }
                      frame True {
                        n239 = property class="CmbBox"(reference=w519) -> (reference out=w521:refnum<vi>, "Strings[]"=w529:string[])  [unwired: 1 in, 1 out]
                        n240 = property class="CmbBox"(reference=w521) -> ("Value"=w520:string)  [unwired: 1 in, 2 out]
                        n241 = while {
                          tunnel: w529 -> [w533] mode=indexing
                          tunnel: [w531] -> w526
                          tunnel: w520 -> [w530]
                          i -> [w531]
                          stop <- w532 stop-if-true
                          n242 = Equal?(x=w533, y=w530) -> (x = y?=w532:bool)
                        }
                        n243 = property class="PmEnumParam"(reference=w528) -> (reference out=w525:refnum<k24>, "Options"=w527:refnum<k24>)  [unwired: 1 in, 1 out]
                        n244 = invoke class="PmReadOnlyObservableCollection`" method="get_Item"(reference=w527, "index"=w526) -> ("get_Item"=w524:refnum<k24>)  [unwired: 2 in, 3 out]
                        n245 = property class="PmEnumItem"(reference=w524) -> ("Value"=w523:i32)  [unwired: 1 in, 2 out]
                        n246 = property class="PmEnumParam"(reference=w525, "Current"=w524) -> ()  [unwired: 1 in, 2 out]
                        n247 = property class="DigNum (strict)"(reference=w522, "Value"=w523) -> ()  [unwired: 1 in, 2 out]
                      }
                    }
                    n248 = case shown="True" w483 {
                      tunnel: w484 -> [_ w513]
                      tunnel: w486 -> [_ w507]
                      tunnel: w485 -> [_ w504]
                      frame False {
                      }
                      frame True {
                        n249 = property class="CmbBox"(reference=w504) -> (reference out=w506:refnum<vi>, "Strings[]"=w514:string[])  [unwired: 1 in, 1 out]
                        n250 = property class="CmbBox"(reference=w506) -> ("Value"=w505:string)  [unwired: 1 in, 2 out]
                        n251 = while {
                          tunnel: w514 -> [w518] mode=indexing
                          tunnel: [w516] -> w511
                          tunnel: w505 -> [w515]
                          i -> [w516]
                          stop <- w517 stop-if-true
                          n252 = Equal?(x=w518, y=w515) -> (x = y?=w517:bool)
                        }
                        n253 = property class="PmEnumParam"(reference=w513) -> (reference out=w510:refnum<k24>, "Options"=w512:refnum<k24>)  [unwired: 1 in, 1 out]
                        n254 = invoke class="PmReadOnlyObservableCollection`" method="get_Item"(reference=w512, "index"=w511) -> ("get_Item"=w509:refnum<k24>)  [unwired: 2 in, 3 out]
                        n255 = property class="PmEnumItem"(reference=w509) -> ("Value"=w508:i32)  [unwired: 1 in, 2 out]
                        n256 = property class="PmEnumParam"(reference=w510, "Current"=w509) -> ()  [unwired: 1 in, 2 out]
                        n257 = property class="DigNum (strict)"(reference=w507, "Value"=w508) -> ()  [unwired: 1 in, 2 out]
                      }
                    }
                    n258 = local read "Exposure Time"() -> (w497:dbl)
                    n259 = In Range and Coerce(upper limit=w502, x=w497, lower limit=w501) -> (coerced(x)=w498:dbl)  [unwired: 1 out]
                    n260 = property class="CameraSettings"(reference=w489, "Exposure"=w498) -> ()  [unwired: 1 in, 2 out]
                    n261 = property class="PmNumericParam`1[[System.UInt64"(reference=w500, "Current"=w498) -> (reference out=w499:refnum<k24>)  [unwired: 1 in, 1 out]
                    n262 = property class="PmNumericParam`1[[System.UInt64"(reference=w499) -> ("Current"=w496:u64)  [unwired: 1 in, 2 out]
                    n263 = local write "Exposure Time"(w496) -> ()
                  }
                }
              }
            }
          }
          event "Get ROI": Value Change {
            n264 = event-data() -> ()  [unwired: 1 in, 6 out]
            n265 = case shown="True" "Get ROI" {
              tunnel: w535 -> [w537 w540]
              tunnel: [w537 w539] -> w534
              frame False {
              }
              frame True {
                n266 = local read "Camera Status"() -> (w538:bool)
                n267 = case shown="True" w538 {
                  tunnel: w540 -> [w542 w546]
                  tunnel: [w542 w543] -> w539
                  frame False {
                    n268 = One Button Dialog(message="Camera is not open") -> ()  [unwired: 1 in, 1 out]
                  }
                  frame True {
                    w551 = 0 items=["Idle", "Capturing"] ("Status")
                    n269 = property class="Camera"(reference=w546) -> (reference out=w545:refnum<k24>, "IsOpen"=w550:bool, "Status"=w552:i32)  [unwired: 1 in, 1 out]
                    n270 = Equal?(x=w550, y=TRUE) -> (x = y?=w548:bool)
                    n271 = Equal?(x=w552, y=w551) -> (x = y?=w547:bool)
                    n272 = Equal?(x=w548, y=w547) -> (x = y?=w544:bool)
                    n273 = case shown="True" w544 {
                      tunnel: w545 -> [w554 w562]
                      tunnel: [w554 w561] -> w543
                      frame False {
                        n274 = One Button Dialog(message="Camera must be idle.") -> ()  [unwired: 1 in, 1 out]
                      }
                      frame True {
                        n275 = property class="Camera"(reference=w562) -> (reference out=w561:refnum<k24>, "Settings"=w560:refnum<k24>)  [unwired: 1 in, 1 out]
                        n276 = property class="CameraSettings"(reference=w560) -> ("Regions"=w559:refnum<k24>)  [unwired: 1 in, 2 out]
                        n277 = property class="PmObservableCollection`1[[PVCam"(reference=w559) -> (reference out=w555:refnum<k24>, "Count"=w558:i32)  [unwired: 1 in, 1 out]
                        n278 = Greater?(x=w558, y=0) -> (0:w556:bool)
                        n279 = case shown="True" w556 {
                          tunnel: w555 -> [_ w564]
                          frame False {
                            n280 = One Button Dialog(message="ROI is not created.") -> ()  [unwired: 1 in, 1 out]
                          }
                          frame True {
                            n281 = invoke class="PmObservableCollection`1[[PVCam" method="get_Item"(reference=w564, "index"=0) -> ("get_Item"=w570:refnum<k24>)  [unwired: 2 in, 3 out]
                            n282 = property class="PmRegion"(reference=w570) -> ("Height"=w568:u16, "Width"=w567:u16, "X"=w566:u16, "Y"=w565:u16)  [unwired: 1 in, 2 out]
                            n283 = local write "Height"(w568) -> ()
                            n284 = local write "Width"(w567) -> ()
                            n285 = local write "X"(w566) -> ()
                            n286 = local write "Y"(w565) -> ()
                          }
                        }
                      }
                    }
                  }
                }
              }
            }
          }
          event "X", "Width", "Y", "Height": Value Change {
            n287 = event-data() -> ()  [unwired: 1 in, 6 out]
            n288 = local read "Camera Status"() -> (w573:bool)
            n289 = case shown="True" w573 {
              tunnel: w572 -> [w574 w577]
              tunnel: [w574 w575] -> w571
              frame False {
              }
              frame True {
                w583 = 0 items=["Idle", "Capturing"] ("Status")
                n290 = property class="Camera"(reference=w577) -> (reference out=w576:refnum<k24>, "IsOpen"=w582:bool, "Status"=w584:i32)  [unwired: 1 in, 1 out]
                n291 = Equal?(x=w582, y=TRUE) -> (x = y?=w580:bool)
                n292 = Equal?(x=w584, y=w583) -> (x = y?=w579:bool)
                n293 = Equal?(x=w580, y=w579) -> (x = y?=w578:bool)
                n294 = case shown="True" w578 {
                  tunnel: w576 -> [w585 w587]
                  tunnel: [w585 w586] -> w575
                  frame False {
                  }
                  frame True {
                    n295 = flat-sequence {
                      tunnel: w587 -> [w635]
                      tunnel: [w634] -> w586
                      frame #0 {
                        # "if (!( x >= 0\n            && (x+width) <= full_width\n            &&  0 < width \n            && y >= 0\n            && (y+height) <= full_height\n            && 0 < height ))\n        {\n           printf(\"Incorrect range for a ROI. \\n\");\n        }"
                        n296 = local read "Width"() -> (w603:u16)
                        n297 = local read "Height"() -> (w601:u16)
                        n298 = local read "Full CCD Height"() -> (w597:u16)
                        n299 = local read "Full CCD Width"() -> (w599:u16)
                        n300 = local read "X"() -> (w604:u16)
                        n301 = local read "Y"() -> (w600:u16)
                        n302 = local read "Height"() -> (w592:u16)
                        n303 = Add(x=w604, y=w603) -> (x+y=w598:u16)
                        n304 = local read "Width"() -> (w595:u16)
                        n305 = Add(x=w601, y=w600) -> (x+y=w596:u16)
                        n306 = local read "X"() -> (w605:u16)
                        n307 = local read "Y"() -> (w602:u16)
                        n308 = Less Or Equal?(x=w596, y=w597) -> (x <= y?=w612:bool)
                        n309 = Less Or Equal?(x=w598, y=w599) -> (x <= y?=w615:bool)
                        n310 = Less?(x=u16 0 ("y"), y=w592) -> (x < y?=w611:bool)
                        n311 = Greater Or Equal?(x=w605, y=u16 0) -> (x >= y?=w616:bool)
                        n312 = Less?(x=u16 0 ("y"), y=w595) -> (x < y?=w614:bool)
                        n313 = Greater Or Equal?(x=w602, y=u16 0) -> (x >= y?=w613:bool)
                        n314 = And(x=w612, y=w611) -> (x .and. y?=w607:bool)
                        n315 = And(x=w616, y=w615) -> (x .and. y?=w610:bool)
                        n316 = And(x=w614, y=w613) -> (x .and. y?=w609:bool)
                        n317 = And(x=w610, y=w609) -> (x .and. y?=w608:bool)
                        n318 = And(x=w608, y=w607) -> (x .and. y?=w606:bool)
                        n319 = case shown="False" w606 {
                          tunnel: [w620 w627] -> w591
                          tunnel: [u16 0 ("X") w626] -> w588
                          tunnel: [u16 0 ("Y") w625] -> w589
                          tunnel: [w621 w624] -> w590
                          frame False {
                            n320 = local read "Full CCD Height"() -> (w621:u16)
                            n321 = local read "Full CCD Width"() -> (w620:u16)
                            n322 = One Button Dialog(message="Wrong ROI ! Resetting to full CCD") -> ()  [unwired: 1 in, 1 out]
                          }
                          frame True {
                            n323 = local read "Height"() -> (w624:u16)
                            n324 = local read "Width"() -> (w627:u16)
                            n325 = local read "X"() -> (w626:u16)
                            n326 = local read "Y"() -> (w625:u16)
                          }
                        }
                        n327 = local write "Width"(w591) -> ()
                        n328 = local write "X"(w588) -> ()
                        n329 = local write "Y"(w589) -> ()
                        n330 = local write "Height"(w590) -> ()
                      }
                      frame #1 {
                        n331 = property class="Camera"(reference=w635) -> (reference out=w634:refnum<k24>, "Settings"=w633:refnum<k24>)  [unwired: 1 in, 1 out]
                        n332 = property class="CameraSettings"(reference=w633) -> ("Regions"=w632:refnum<k24>)  [unwired: 1 in, 2 out]
                        n333 = property class="PmObservableCollection`1[[PVCam"(reference=w632) -> (reference out=w628:refnum<k24>, "Count"=w631:i32)  [unwired: 1 in, 1 out]
                        n334 = Greater?(x=w631, y=0) -> (0:w629:bool)
                        n335 = case shown="True" w629 {
                          tunnel: w628 -> [_ w641]
                          frame False {
                            n336 = One Button Dialog(message="ROI is not created.") -> ()  [unwired: 1 in, 1 out]
                          }
                          frame True {
                            n337 = invoke class="PmObservableCollection`1[[PVCam" method="get_Item"(reference=w641, "index"=0) -> ("get_Item"=w643:refnum<k24>)  [unwired: 2 in, 3 out]
                            n338 = local read "Height"() -> (w640:u16)
                            n339 = local read "Width"() -> (w639:u16)
                            n340 = local read "X"() -> (w638:u16)
                            n341 = local read "Y"() -> (w637:u16)
                            n342 = property class="PmRegion"(reference=w643, "Height"=w640, "Width"=w639, "X"=w638, "Y"=w637) -> ()  [unwired: 1 in, 2 out]
                          }
                        }
                      }
                    }
                  }
                }
              }
            }
          }
          event "Full CCD": Value Change {
            n343 = event-data() -> ()  [unwired: 1 in, 6 out]
            n344 = case shown="True" "Full CCD" {
              tunnel: w645 -> [w647 w650]
              tunnel: [w647 w649] -> w644
              frame False {
              }
              frame True {
                n345 = local read "Camera Status"() -> (w648:bool)
                n346 = case shown="True" w648 {
                  tunnel: w650 -> [w652 w656]
                  tunnel: [w652 w653] -> w649
                  frame False {
                    n347 = One Button Dialog(message="Camera is not open") -> ()  [unwired: 1 in, 1 out]
                  }
                  frame True {
                    w661 = 0 items=["Idle", "Capturing"] ("Status")
                    n348 = property class="Camera"(reference=w656) -> (reference out=w655:refnum<k24>, "IsOpen"=w660:bool, "Status"=w662:i32)  [unwired: 1 in, 1 out]
                    n349 = Equal?(x=w660, y=TRUE) -> (x = y?=w658:bool)
                    n350 = Equal?(x=w662, y=w661) -> (x = y?=w657:bool)
                    n351 = Equal?(x=w658, y=w657) -> (x = y?=w654:bool)
                    n352 = case shown="True" w654 {
                      tunnel: w655 -> [w663 w672]
                      tunnel: [w663 w671] -> w653
                      frame False {
                      }
                      frame True {
                        n353 = property class="Camera"(reference=w672) -> (reference out=w671:refnum<k24>, "Settings"=w670:refnum<k24>)  [unwired: 1 in, 1 out]
                        n354 = property class="CameraSettings"(reference=w670) -> (reference out=w664:refnum<k24>, "Regions"=w665:refnum<k24>)  [unwired: 1 in, 1 out]
                        n355 = property class="PmObservableCollection`1[[PVCam"(reference=w665) -> (reference out=w666:refnum<k24>, "Count"=w669:i32)  [unwired: 1 in, 1 out]
                        n356 = Greater?(x=w669, y=0) -> (0:w667:bool)
                        n357 = case shown="True" w667 {
                          tunnel: w666 -> [_ _]
                          tunnel: w665 -> [_ w681]
                          tunnel: w664 -> [_ w675]
                          frame False {
                          }
                          frame True {
                            n358 = invoke class="PmObservableCollection`1[[PVCam" method="RemoveAt"(reference=w681, "index"=0) -> ()  [unwired: 2 in, 4 out]
                            n359 = property class="CameraSettings"(reference=w675) -> ("SensorWidth"=w677:refnum<k24>)  [unwired: 1 in, 2 out]
                            n360 = property class="CameraSettings"(reference=w675) -> ("SensorHeight"=w678:refnum<k24>)  [unwired: 1 in, 2 out]
                            n361 = property class="PmNumericParam`1[[System.UInt32"(reference=w677) -> ("Current"=w676:u32)  [unwired: 1 in, 2 out]
                            n362 = property class="PmNumericParam`1[[System.UInt32"(reference=w678) -> ("Current"=w679:u32)  [unwired: 1 in, 2 out]
                            n363 = local write "Y"(0 ("index")) -> ()
                            n364 = local write "Width"(w676) -> ()
                            n365 = local write "Height"(w679) -> ()
                            n366 = local write "X"(0 ("index")) -> ()
                          }
                        }
                      }
                    }
                  }
                }
              }
            }
          }
          event "Live start": Value Change {
            n367 = event-data() -> ()  [unwired: 1 in, 6 out]
            n368 = case shown="True" "Live start" {
              tunnel: w684 -> [w686 w689]
              tunnel: [w686 w688] -> w683
              frame False {
              }
              frame True {
                n369 = local read "Camera Status"() -> (w687:bool)
                n370 = case shown="True" w687 {
                  tunnel: w689 -> [w690 w695]
                  tunnel: [w690 w693] -> w688
                  frame False {
                    n371 = One Button Dialog(message="Camera is not open") -> ()  [unwired: 1 in, 1 out]
                  }
                  frame True {
                    w700 = 0 items=["Idle", "Capturing"] ("Status")
                    n372 = property class="Camera"(reference=w695) -> (reference out=w694:refnum<k24>, "IsOpen"=w699:bool, "Status"=w701:i32)  [unwired: 1 in, 1 out]
                    n373 = Equal?(x=w699, y=TRUE) -> (x = y?=w697:bool)
                    n374 = Equal?(x=w701, y=w700) -> (x = y?=w696:bool)
                    n375 = Equal?(x=w697, y=w696) -> (x = y?=w692:bool)
                    n376 = case shown="True" w692 {
                      tunnel: w694 -> [w703 w705]
                      tunnel: [w703 w706] -> w693
                      frame False {
                        n377 = local write "Live"(FALSE ("Live 2")) -> ()
                      }
                      frame True {
                        n378 = flat-sequence {
                          tunnel: w705 -> [w711]
                          tunnel: [w708] -> w704
                          frame #0 {
                            n379 = property class="Camera"(reference=w711) -> (reference out=w708:refnum<k24>, "AcquisitionBuffer"=w710:refnum<k24>)  [unwired: 1 in, 1 out]
                            n380 = property class="AcqBuffer"(reference=w710, "BufferSize"=100) -> ()  [unwired: 1 in, 2 out]
                          }
                        }
                        n381 = local write "Live"(TRUE ("Live")) -> ()
                        n382 = invoke class="Camera" method="StartLive"(reference=w704) -> (reference out=w706:refnum<k24>)  [unwired: 2 in, 2 out]
                      }
                    }
                  }
                }
              }
            }
          }
          event "Live stop": Value Change {
            n383 = event-data() -> ()  [unwired: 1 in, 6 out]
            n384 = case shown="True" "Live stop" {
              tunnel: w713 -> [w715 w718]
              tunnel: [w715 w717] -> w712
              frame False {
              }
              frame True {
                n385 = local read "Camera Status"() -> (w716:bool)
                n386 = case shown="False" w716 {
                  tunnel: w718 -> [w720 w730]
                  tunnel: [w720 w727] -> w717
                  frame False {
                    n387 = One Button Dialog(message="Camera is not open") -> ()  [unwired: 1 in, 1 out]
                  }
                  frame True {
                    w725 = 1 items=["Idle", "Capturing"] ("Status")
                    n388 = property class="Camera"(reference=w730) -> (reference out=w728:refnum<k24>, "IsOpen"=w724:bool, "Status"=w726:i32)  [unwired: 1 in, 1 out]
                    n389 = Equal?(x=w726, y=w725) -> (x = y?=w721:bool)
                    n390 = Equal?(x=w724, y=TRUE) -> (x = y?=w722:bool)
                    n391 = Equal?(x=w722, y=w721) -> (x = y?=w729:bool)
                    n392 = case shown="True" w729 {
                      tunnel: w728 -> [w731 w734]
                      tunnel: [w731 w733] -> w727
                      frame False {
                      }
                      frame True {
                        n393 = invoke class="Camera" method="Stop"(reference=w734) -> (reference out=w733:refnum<k24>)  [unwired: 2 in, 2 out]
                        n394 = local write "Live"(FALSE ("Live 2")) -> ()
                      }
                    }
                  }
                }
              }
            }
          }
          event "Uninit": Value Change {
            n395 = event-data() -> ()  [unwired: 1 in, 6 out]
            n396 = case shown="True" "Uninit" {
              tunnel: w739 -> [w741 w745]
              tunnel: [w741 w744] -> w738
              tunnel: [FALSE ("Camera Status") w742] -> w736
              frame False {
              }
              frame True {
                n397 = local read "Camera Status"() -> (w743:bool)
                n398 = case shown="True" w743 {
                  tunnel: w745 -> [w747 w752]
                  tunnel: [w747 w751] -> w744
                  tunnel: [FALSE ("Camera Status") w750] -> w742
                  frame False {
                  }
                  frame True {
                    n399 = local read "Live"() -> (w748:bool)
                    n400 = Not(x=w748) -> (.not. x?=w749:bool)
                    n401 = case shown="True" w749 {
                      tunnel: w752 -> [w754 w757]
                      tunnel: [w754 w756] -> w751
                      tunnel: [FALSE ("Camera Status") w755] -> w750
                      frame False {
                      }
                      frame True {
                        n402 = flat-sequence {
                          tunnel: w757 -> [w760]
                          tunnel: [w759] -> w758
                          tunnel: [w763] -> w756
                          tunnel: w758 -> [w763]
                          tunnel: [TRUE ("Camera Status")] -> w755
                          frame #0 {
                            n403 = invoke class="Camera" method="Close"(reference=w760) -> (reference out=w759:refnum<k24>)  [unwired: 2 in, 2 out]
                          }
                          frame #1 {
                            n404 = local write "Camera Status"(FALSE ("Camera Status")) -> ()
                          }
                        }
                      }
                    }
                  }
                }
              }
            }
          }
        }
      }
    }
    frame #2 {
      n405 = invoke class="Library" method="Release"(reference=w765) -> (reference out=w766:refnum<k24>)  [unwired: 2 in, 2 out]
      n406 = Wait (ms)(milliseconds to wait=u32 100) -> ()  [unwired: 1 out]
      n407 = Close Reference(reference=w766) -> ()  [unwired: 1 in, 1 out]
    }
    frame #3 {
      n408 = invoke class="GC" method="Collect"() -> ()  [unwired: 3 in, 3 out]
    }
  }
  n409 = control-ref of="Exp. out"() -> (w3:refnum<vi>)
  n410 = property class="DigNum (strict)"(reference=w3, "Visible"=FALSE) -> ()  [unwired: 1 in, 2 out]
  n411 = control-ref of="Trigger Mode"() -> (w2:refnum<vi>)
  n412 = property class="DigNum (strict)"(reference=w2, "Visible"=FALSE) -> ()  [unwired: 1 in, 2 out]
  n413 = control-ref of="Trigger Out Behaviour"() -> (w8:refnum<vi>)
  n414 = control-ref of="Exp. out"() -> (w6:refnum<vi>)
  n415 = property class="DigNum (strict)"(reference=w6, "Value"=0) -> ()  [unwired: 1 in, 2 out]
  n416 = property class="CmbBox"(reference=w8, "Value"="") -> ()  [unwired: 1 in, 2 out]
  n417 = local write "Camera Status"(FALSE ("Camera Status")) -> ()
  n418 = property on="Scan Width" class="DigNum (strict)"("DisabledEnum"=w11) -> ()  [unwired: 2 in, 2 out]
  n419 = property on="Scan Line Delay" class="DigNum (strict)"("DisabledEnum"=w11) -> ()  [unwired: 2 in, 2 out]
  n420 = control-ref of="Scan Line Delay"() -> (w14:refnum<vi>)
  n421 = control-ref of="Scan Width"() -> (w17:refnum<vi>)
  n422 = control-ref of="Scan Line Time"() -> (w13:refnum<vi>)
  n423 = control-ref of="Scan Direction"() -> (w20:refnum<vi>)
  n424 = control-ref of="Scan Mode"() -> (w23:refnum<vi>)
  n425 = property class="CmbBox"(reference=w23, "Value"="", "Strings[]"=string[] [] ("Strings []")) -> ()  [unwired: 1 in, 2 out]
  n426 = property class="DigNum (strict)"(reference=w14, "Value"=0.0) -> ()  [unwired: 1 in, 2 out]
  n427 = property class="CmbBox"(reference=w20, "Strings[]"=string[] [] ("Strings []"), "Value"="") -> ()  [unwired: 1 in, 2 out]
  n428 = property class="DigNum (strict)"(reference=w17, "Value"=0.0) -> ()  [unwired: 1 in, 2 out]
  n429 = property class="DigNum (strict)"(reference=w13, "Value"=0.0) -> ()  [unwired: 1 in, 2 out]
  n430 = local write "Scan Direction Reset"(FALSE ("Boolean")) -> ()
  "Boolean" <- FALSE ("Boolean")
